vi "Set Default Values.vi"(8 "error in (no error)":errorcluster, 11 "User Interface in":refnum<class "User Interface.lvclass">) -> (0 "error out":errorcluster, 3 "User Interface out":refnum<class "User Interface.lvclass">)   [LabVIEW 2015, in "User Interface.lvlib" / "User Interface.lvclass"]
uses:
  User Interface.lvclass
  User Interface.lvclass/User Interface.ctl
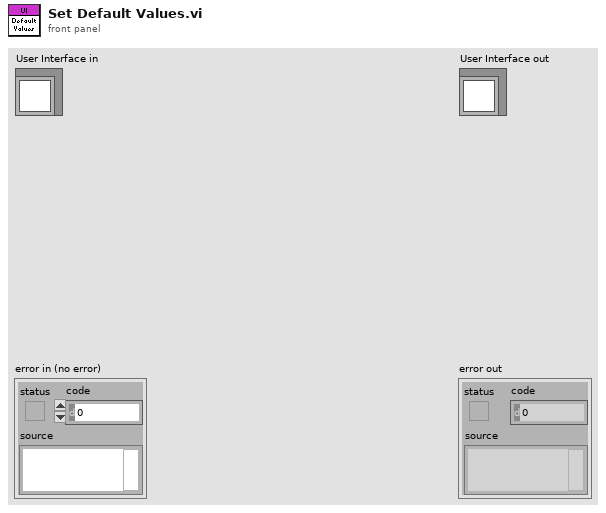
[diagram p1: front panel]
types:
  T1 = enum8{"Enabled", "Disabled", "Disabled and Grayed Out"}
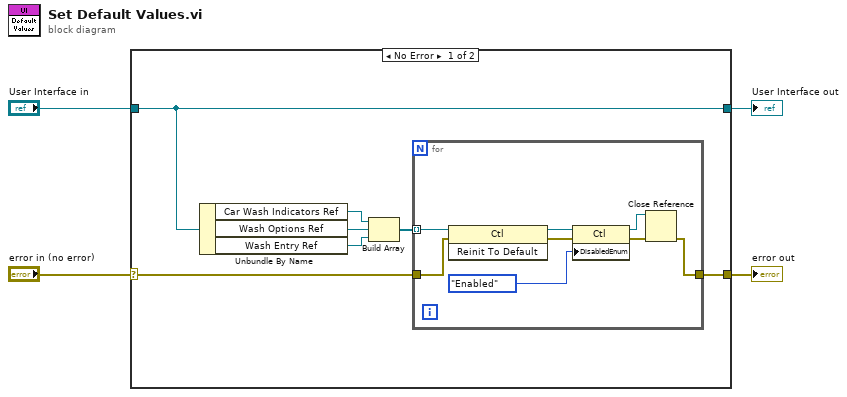
[diagram p0: block diagram]
diagram:
  n1 = case shown="No Error" "error in (no error)" {
    selector: "error in (no error)" -> [w6 w21]
    tunnel: [w5 w21] -> w3
    tunnel: [w11 w20] -> w1
    tunnel: "User Interface in" -> [w11 w20]
    frame No Error {
      n2 = Unbundle By Name(w11) -> ("Car Wash Indicators Ref"=w10:refnum<vi>, "Wash Options Ref"=w9:refnum<vi>, "Wash Entry Ref"=w8:refnum<vi>)
      n3 = Build Array(w10, w9, w8) -> (w7:refnum<vi>[])
      n4 = for {
        tunnel: w7 -> [w19] mode=indexing
        tunnel: w6 -> [w15]
        tunnel: [w12] -> w5
        n5 = invoke class="Ctl" method="Reinit To Default"(reference=w19, error in=w15) -> (reference out=w18:refnum<vi>, error out=w17:errorcluster)  [unwired: 1 in, 1 out]
        n6 = property class="Ctl"(reference=w18, error in=w17, "DisabledEnum"=T1."Enabled" ("Disabled")) -> (reference out=w13:refnum<vi>, error out=w14:errorcluster)
        n7 = Close Reference(reference=w13, error in (no error)=w14) -> (error out=w12:errorcluster)
      }
    }
    frame Error {
    }
  }
  "error out" <- w3
  "User Interface out" <- w1
